vi "polynomal curve fitting2015.vi"() -> ()   [LabVIEW 2015]
uses:
  <vilib>/Analysis/NI_AALPro.lvlib
  <vilib>/Utility/file.llb/Read Delimited Spreadsheet (DBL).vi
panel:
  in  "Polynomial Degree 3":dbl
  out "Waveform Graph 3":dbl[](graph)
  in  "Polynomial Degree 2":dbl
  out "Waveform Graph 2":dbl[](graph)
  out "Prepared by \nthe project":string
  in  "Polynomial Degree":dbl
  out "Waveform Graph":dbl[](graph)
  out "Data":dbl[][](array[numeric])
  in  "Measurement file \nwith extension Txt":path
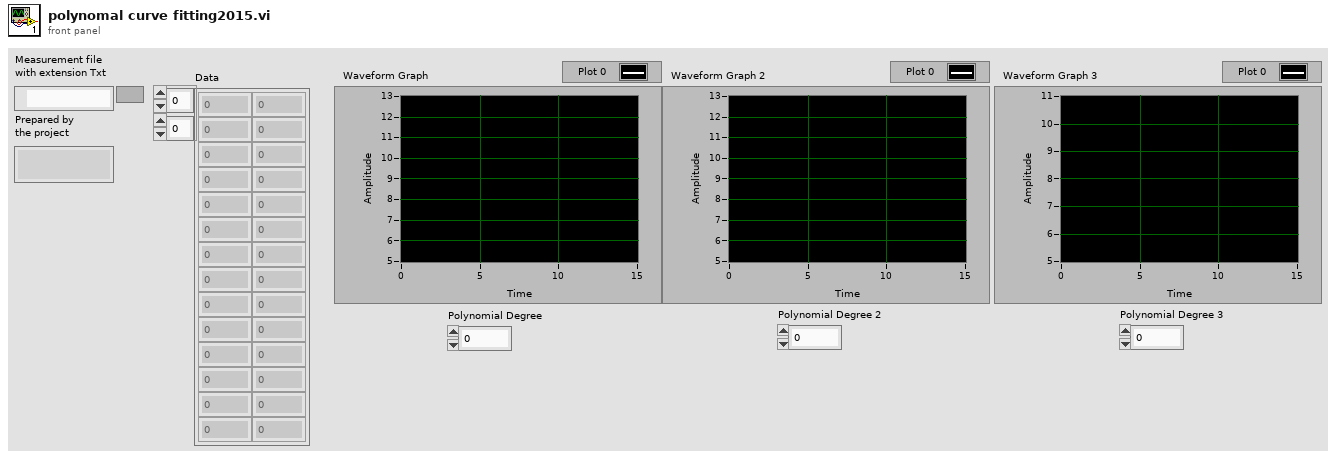
[diagram p1: front panel]
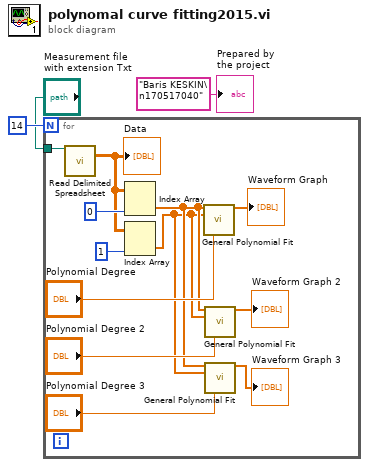
[diagram p0: block diagram]
diagram:
  n1 = for {
    N: 14 -> [_]
    tunnel: "Measurement file \nwith extension Txt" -> [w15]
    n2 = call-poly <vilib>:"Read Delimited Spreadsheet.vi"("file path (dialog if empty)"=w15) -> ("all rows"=w12:dbl[][])  [unwired: 9 in, 5 out]
    "Data" <- w12
    n3 = Index Array(array=w12, index (col)=0 ("disabled index (col)")) -> (element=w5:dbl[])  [unwired: 1 in]
    n4 = Index Array(array=w12, index (col)=1 ("disabled index (col)")) -> (element=w4:dbl[])  [unwired: 1 in]
    n5 = call <vilib>:"General Polynomial Fit.vi"("Y"=w5, "polynomial order"="Polynomial Degree", "X"=w4) -> ("Best Polynomial Fit"=→"Waveform Graph":dbl[])  [unwired: 9 in, 3 out]
    n6 = call <vilib>:"General Polynomial Fit.vi"("Y"=w5, "polynomial order"="Polynomial Degree 2", "X"=w4) -> ("Best Polynomial Fit"=→"Waveform Graph 2":dbl[])  [unwired: 9 in, 3 out]
    n7 = call <vilib>:"General Polynomial Fit.vi"("Y"=w5, "polynomial order"="Polynomial Degree 3", "X"=w4) -> ("Best Polynomial Fit"=→"Waveform Graph 3":dbl[])  [unwired: 9 in, 3 out]
  }
  "Prepared by \nthe project" <- "Baris KESKIN\n170517040"
